vi "GetQueueRef.vi"(6 "GetQueueRef":T1, 8 "error in (no error)":errorcluster, 10 "SubsystemData.lvclass":refnum<class "SubsystemData.lvclass">, 11 "Subsystem in":refnum<class "Subsystem.lvclass">) -> (0 "error out":errorcluster, 3 "Subsystem out":refnum<class "Subsystem.lvclass">)   [LabVIEW 2017, in "Subsystem.lvclass"]
uses:
  Subsystem.lvclass
  SubsystemData/SubsystemData.lvclass
  GetQueueRef.ctl
  Subsystem.lvclass/Subsystem.ctl
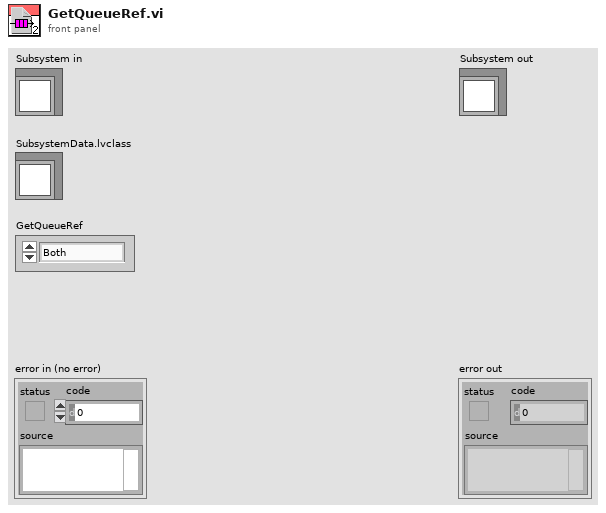
[diagram p1: front panel]
types:
  T1 = typedef "Subsystem.lvclass/GetQueueRef.ctl" = enum16{"Both", "Command", "Output"}
  T2 = typedef "SubsystemData.lvclass/GenericData.ctl" = cluster{"Subsystem Name":string, "Command Origin":T3}
  T3 = typedef "SubsystemData.lvclass/CommandOrigin.ctl" = enum16{"Teleop", "Auto"}
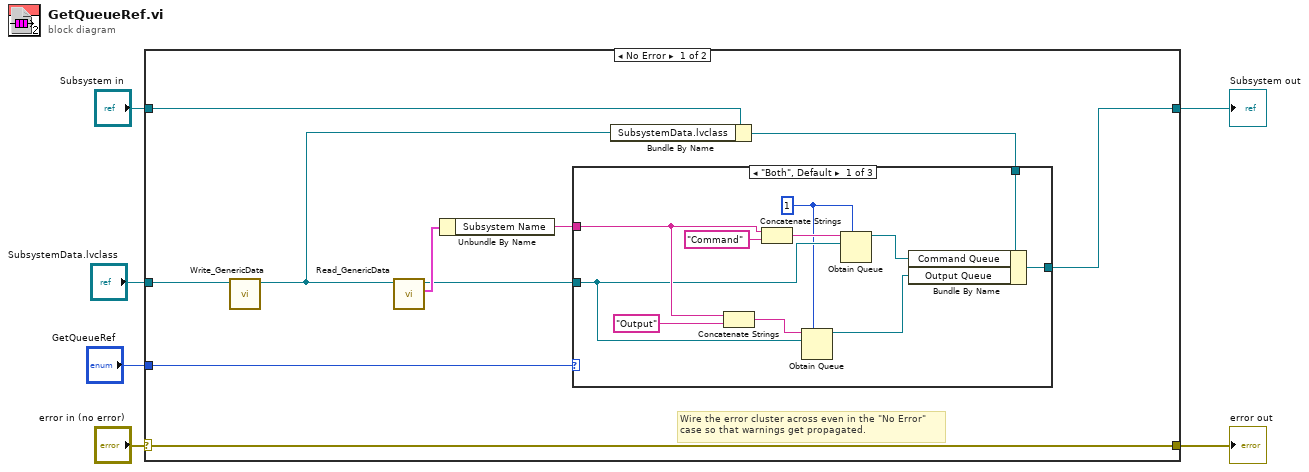
[diagram p0: block diagram]
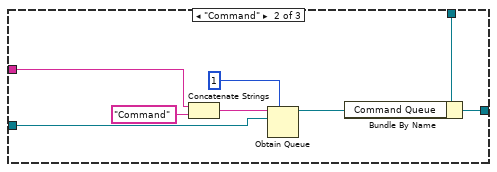
[diagram p2: hidden frame]
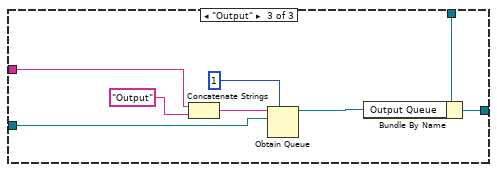
[diagram p3: hidden frame]
diagram:
  n1 = case shown="No Error" "error in (no error)" {
    selector: "error in (no error)" -> [w16 w45]
    tunnel: [w16 w45] -> w5
    tunnel: [w11 w44] -> w2
    tunnel: "Subsystem in" -> [w10 w44]
    tunnel: "SubsystemData.lvclass" -> [w8 _]
    tunnel: "GetQueueRef" -> [w12 _]
    frame No Error {
      # "Wire the error cluster across even in the \"No Error\"\ncase so that warnings get propagated."
      n2 = call-dynamic "Write_GenericData.vi"("SubsystemData in"=w8) -> ("SubsystemData out"=w7:refnum<class "SubsystemData.lvclass">)  [unwired: 9 in, 1 out]
      n3 = call-dynamic "Read_GenericData.vi"("SubsystemData in"=w7) -> ("Data"=w15:T2, "SubsystemData out"=w13:refnum<class "SubsystemData.lvclass">)  [unwired: 8 in, 1 out]
      n4 = Unbundle By Name(w15) -> ("Subsystem Name"=w14:string)
      n5 = Bundle By Name(cluster=w10, "SubsystemData.lvclass"=w7) -> (w9:refnum<class "Subsystem.lvclass">)
      n6 = case shown="\"Both\", Default" w12 {
        tunnel: w14 -> [w23 w31 w39]
        tunnel: w13 -> [w22 w30 w38]
        tunnel: w9 -> [w21 w29 w37]
        tunnel: [w20 w28 w36] -> w11
        frame "Both", Default {
          w17 = 1 ("max queue size (-1, unlimited)")
          n7 = Concatenate Strings(w23, "Output") -> (w24:string)
          n8 = Concatenate Strings(w23, "Command") -> (w26:string)
          n9 = Obtain Queue(max queue size (-1, unlimited)=w17, name (unnamed)=w24, element data type=w22) -> (queue out=w18:refnum<queue>)  [unwired: 2 in, 2 out]
          n10 = Obtain Queue(max queue size (-1, unlimited)=w17, name (unnamed)=w26, element data type=w22) -> (queue out=w19:refnum<queue>)  [unwired: 2 in, 2 out]
          n11 = Bundle By Name(cluster=w21, "Command Queue"=w19, "Output Queue"=w18) -> (w20:refnum<class "Subsystem.lvclass">)
        }
        frame "Command" {
          n12 = Concatenate Strings(w31, "Command") -> (w34:string)
          n13 = Obtain Queue(max queue size (-1, unlimited)=1, name (unnamed)=w34, element data type=w30) -> (queue out=w32:refnum<queue>)  [unwired: 2 in, 2 out]
          n14 = Bundle By Name(cluster=w29, "Command Queue"=w32) -> (w28:refnum<class "Subsystem.lvclass">)
        }
        frame "Output" {
          n15 = Concatenate Strings(w39, "Output") -> (w42:string)
          n16 = Obtain Queue(max queue size (-1, unlimited)=1, name (unnamed)=w42, element data type=w38) -> (queue out=w40:refnum<queue>)  [unwired: 2 in, 2 out]
          n17 = Bundle By Name(cluster=w37, "Output Queue"=w40) -> (w36:refnum<class "Subsystem.lvclass">)
        }
      }
    }
    frame Error {
    }
  }
  "error out" <- w5
  "Subsystem out" <- w2
